vi "Calculadora.vi"(9 "y":dbl format="%#_13g", 10 "x":dbl format="%#_13g", 11 "Operacion":T1(ring)) -> (3 "Resultado":dbl)   [LabVIEW 2024]
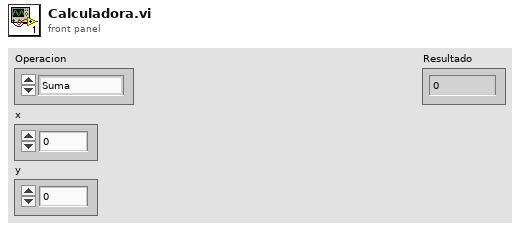
[diagram p1: front panel]
types:
  T1 = enum16{"Suma", "Resta", "Multiplicacion", "Division"}
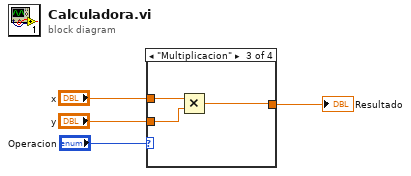
[diagram p0: block diagram]
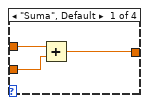
[diagram p2: hidden frame]
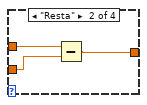
[diagram p3: hidden frame]
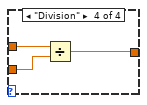
[diagram p4: hidden frame]
diagram:
  n1 = case shown="\"Multiplicacion\"" "Operacion" {
    tunnel: "x" -> [w7 w10 w13 w16]
    tunnel: "y" -> [w6 w9 w12 w15]
    tunnel: [w5 w8 w11 w14] -> w1
    frame "Suma", Default {
      n2 = Add(x=w7, y=w6) -> (x+y=w5:dbl)
    }
    frame "Resta" {
      n3 = Subtract(x=w10, y=w9) -> (x-y=w8:dbl)
    }
    frame "Multiplicacion" {
      n4 = Multiply(x=w13, y=w12) -> (x*y=w11:dbl)
    }
    frame "Division" {
      n5 = Divide(x=w16, y=w15) -> (x/y=w14:dbl)
    }
  }
  "Resultado" <- w1
